vi "Complex To Polar - CM.vi"(0 "Complex Matrix r*e^iQ":T2) -> (1 "Modulus r":T1, 2 "Argument Q":T1)   [LabVIEW 2018, in "NI_Matrix.lvlib"]
doc: "Breaks a complex number into its polar components."
uses:
  NI_Matrix.lvlib
  ComplexMatrix.ctl
  RealMatrix.ctl
  Matrix To Array - CM.vi
  Array To Matrix - RA2.vi
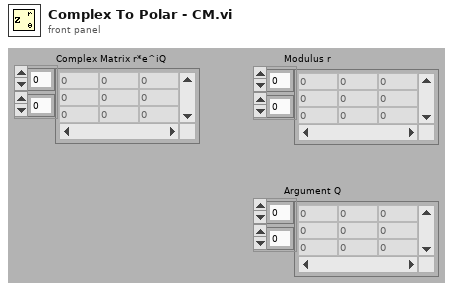
[diagram p1: front panel]
types:
  T1 = typedef "NI_Matrix.lvlib/RealMatrix.ctl" = dbl[][]
  T2 = typedef "NI_Matrix.lvlib/ComplexMatrix.ctl" = cdb[][]
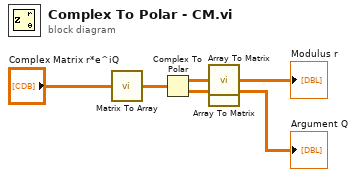
[diagram p0: block diagram]
diagram:
  n1 = call-poly "Matrix To Array.vi"("Complex Matrix"="Complex Matrix r*e^iQ") -> ("Complex 2D Array"=w6:cdb[][])
  n2 = Complex To Polar(r * e^(i*theta)=w6) -> (r=w4:dbl[][], theta=w2:dbl[][])
  n3 = call-poly "Array To Matrix.vi"("Real 2D Array"=w4) -> ("Real Matrix"=→"Modulus r":T1)
  n4 = call-poly "Array To Matrix.vi"("Real 2D Array"=w2) -> ("Real Matrix"=→"Argument Q":T1)
